vi "Coerce Pixels per Unit.vi"(11 "pixels per unit":dbl) -> (3 "coerced pixels per unit":dbl)   [LabVIEW 2017, in "NI_Robotics_Configure Steering Frame.lvlib"]
uses:
  <vilib>/robotics/Dialog/Configure Steering Frame/NI_Robotics_Configure Steering Frame.lvlib
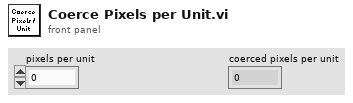
[diagram p1: front panel]
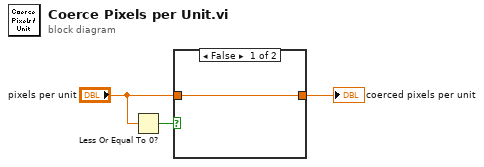
[diagram p0: block diagram]
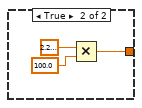
[diagram p2: hidden frame]
diagram:
  n1 = Less Or Equal To 0?(x="pixels per unit") -> (x <= 0?=w3:bool)
  n2 = case shown="False" w3 {
    tunnel: "pixels per unit" -> [w4 _]
    tunnel: [w4 w5] -> w1
    frame False {
    }
    frame True {
      n3 = Multiply(x=2.220446049250313e-16, y=100.0) -> (x*y=w5:dbl)
    }
  }
  "coerced pixels per unit" <- w1
